vi "New Credit and cambio to Dinero.vi"(8 "error in (no error)":errorcluster, 9 "Cambio":i32, 10 "Credito":i32, 11 "UI in":refnum<class "UI.lvclass">) -> (0 "error out":errorcluster, 3 "UI out":refnum<class "UI.lvclass">)   [LabVIEW 2020, in "UI.lvlib" / "UI.lvclass"]
uses:
  UI.lvclass
  UI.lvclass/UI.ctl
  Dinero Messages/Obtain New Credit and cambio from UI Msg/Obtain New Credit and cambio from UI Msg.lvclass/Obtain New Credit and cambio from UI Msg.ctl
  <vilib>/ActorFramework/Message Enqueuer/Message Enqueuer.lvclass/Message Enqueuer.ctl
  <vilib>/ActorFramework/Message Enqueuer/Enqueue.vi
  Dinero Messages/Obtain New Credit and cambio from UI Msg/Obtain New Credit and cambio from UI Msg.lvclass
  C:/Program Files (x86)/National Instruments/LabVIEW 2020/vi.lib/ActorFramework/Message/Message.lvclass
  <vilib>/ActorFramework/Message Priority Queue/Priority Enqueue.vi
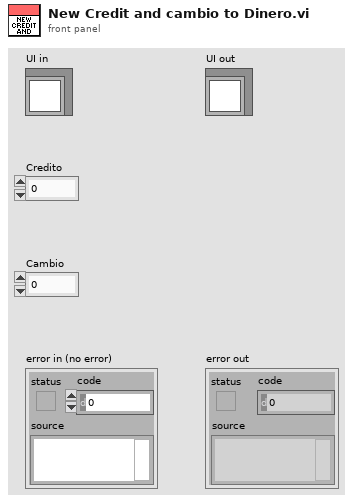
[diagram p1: front panel]
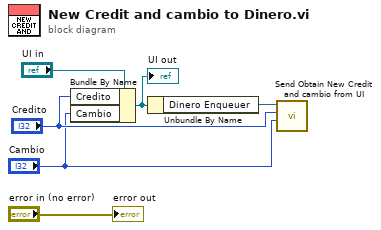
[diagram p0: block diagram]
diagram:
  n1 = Bundle By Name(cluster="UI in", "Credito"="Credito", "Cambio"="Cambio") -> (w4:refnum<class "UI.lvclass">)
  "UI out" <- w4
  n2 = Unbundle By Name(w4) -> ("Dinero Enqueuer"=w3:refnum<class "Message Enqueuer.lvclass">)
  n3 = call "Send Obtain New Credit and cambio from UI.vi"("Cambio"="Cambio", "Credito"="Credito", "Message Enqueuer"=w3) -> ()  [unwired: 7 in, 2 out]
  "error out" <- "error in (no error)"
